vi "getObjectRefs.vi"(8 "error in (no error)":errorcluster, 11 "Structure in":refnum<class "Structure.lvclass">) -> (0 "error out":errorcluster, 3 "Structure out":refnum<class "Structure.lvclass">)   [LabVIEW 2023, in "TLC_Scripto.lvlib" / "Structure.lvclass"]
uses:
  Structure.lvclass
  Structure.lvclass/Structure.ctl
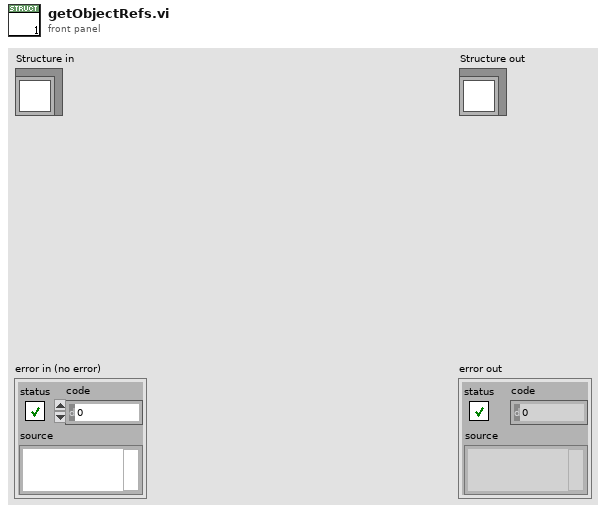
[diagram p1: front panel]
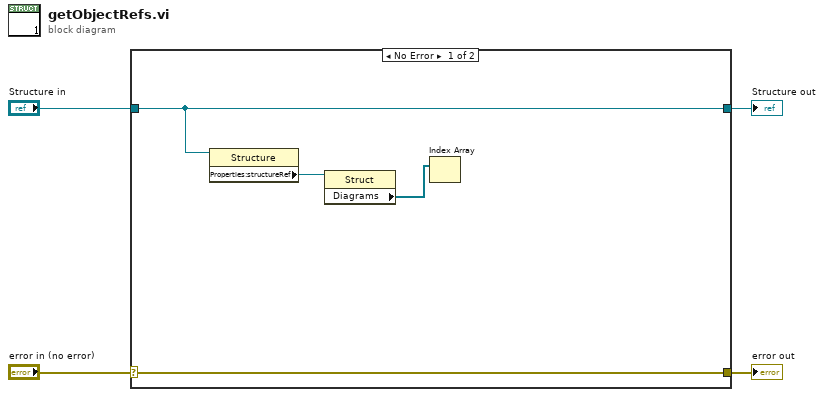
[diagram p0: block diagram]
diagram:
  n1 = case shown="No Error" "error in (no error)" {
    selector: "error in (no error)" -> [w8 w10]
    tunnel: [w8 w10] -> w3
    tunnel: [w7 w9] -> w1
    tunnel: "Structure in" -> [w7 w9]
    frame No Error {
      n2 = property class="Structure"(reference=w7) -> ("Properties:structureRef"=w6:refnum<vi>)  [unwired: 1 in, 2 out]
      n3 = property class="Struct"(reference=w6) -> ("Diagrams"=w5:refnum<vi>[])  [unwired: 1 in, 2 out]
      n4 = Index Array(array=w5) -> ()  [unwired: 1 in, 1 out]
    }
    frame Error {
    }
  }
  "error out" <- w3
  "Structure out" <- w1
